vi "categoryExists.vi"(8 "error in (no error)":errorcluster, 10 "Category.lvclass":refnum<class "Category.lvclass">, 11 "Account History in":refnum<class "Account History.lvclass">) -> (0 "error out":errorcluster, 2 "Exist?":bool, 3 "Account History out":refnum<class "Account History.lvclass">)   [LabVIEW 2018, in "Account History.lvclass"]
uses:
  Account History.lvclass
  Category/Category.lvclass
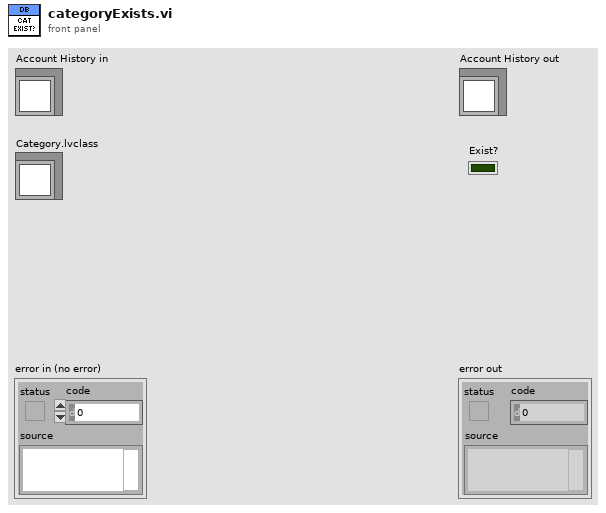
[diagram p1: front panel]
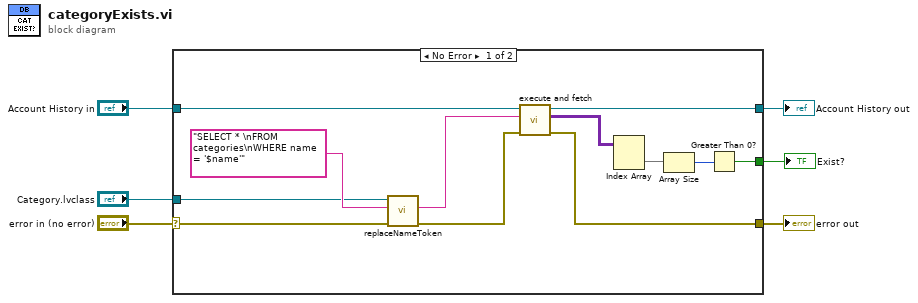
[diagram p0: block diagram]
diagram:
  n1 = case shown="No Error" "error in (no error)" {
    selector: "error in (no error)" -> [w10 w20]
    tunnel: [w16 w20] -> w5
    tunnel: [w17 w19] -> w3
    tunnel: "Account History in" -> [w18 w19]
    tunnel: [w12 _] -> w2
    tunnel: "Category.lvclass" -> [w7 _]
    frame No Error {
      n2 = call "replaceNameToken.vi"("error in (no error)"=w10, "Query In"="SELECT * \nFROM categories\nWHERE name = '$name'", "Category in"=w7) -> ("error out"=w9:errorcluster, "Query Out"=w11:string)  [unwired: 6 in, 1 out]
      n3 = call "execute and fetch.vi"("error in (no error)"=w9, "SQL query"=w11, "Database in"=w18) -> ("error out"=w16:errorcluster, "recordset data"=w15:variant[][], "Database out"=w17:refnum<class "Account History.lvclass">)  [unwired: 5 in, 1 out]
      n4 = Index Array(array=w15) -> (element=w14:variant[])  [unwired: 2 in]
      n5 = Array Size(array=w14) -> (size(s)=w13:i32)
      n6 = Greater Than 0?(x=w13) -> (x > 0?=w12:bool)
    }
    frame Error {
    }
  }
  "error out" <- w5
  "Account History out" <- w3
  "Exist?" <- w2
